vi "Write.vi"(10 "I32 Array":i32[](array[numeric]), 11 "I32 Array in":refnum<class "I32 Array.lvclass">) -> (3 "I32 Array out":refnum<class "I32 Array.lvclass">)   [LabVIEW 2020, in "Data.lvlib" / "I32 Array.lvclass"]
doc: "Write I32 Array."
uses:
  I32 Array.lvclass
  I32 Array.lvclass/I32 Array.ctl
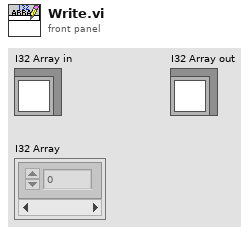
[diagram p1: front panel]
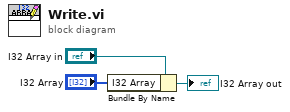
[diagram p0: block diagram]
diagram:
  n1 = Bundle By Name(cluster="I32 Array in", "I32 Array"="I32 Array") -> (→"I32 Array out":refnum<class "I32 Array.lvclass">)
